vi "Read IL Action.vi"(11 "IL Action in":refnum<class "IL Action.lvclass">) -> (1 "Message Priority (Normal)":T1=enum."Normal", 3 "IL Action out":refnum<class "IL Action.lvclass">, 4 "Actor Framework:Message":refnum<class "Message.lvclass">, 5 "Action Destination":refnum<class "Message Enqueuer.lvclass">)   [LabVIEW 2015, in "Interlocks.lvlib" / "IL Action.lvclass"]
uses:
  IL Action.lvclass
  <vilib>/ActorFramework/Message/Message.lvclass
  <vilib>/ActorFramework/Message Enqueuer/Message Enqueuer.lvclass
  <vilib>/ActorFramework/Message Enqueuer/Message Priority.ctl
  IL Action.lvclass/IL Action.ctl
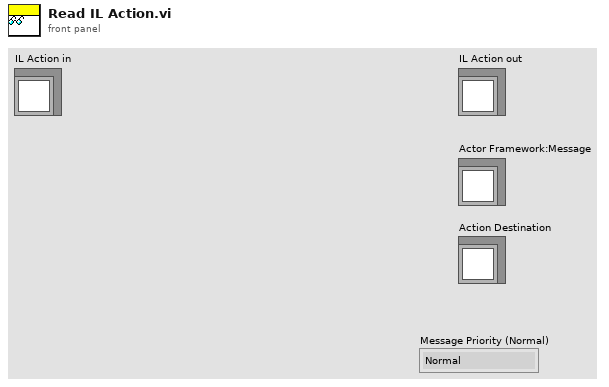
[diagram p1: front panel]
types:
  T1 = typedef "Actor Framework.lvlib/Message Enqueuer.lvclass/Message Priority.ctl" = enum16{"Low", "Normal", "High"}
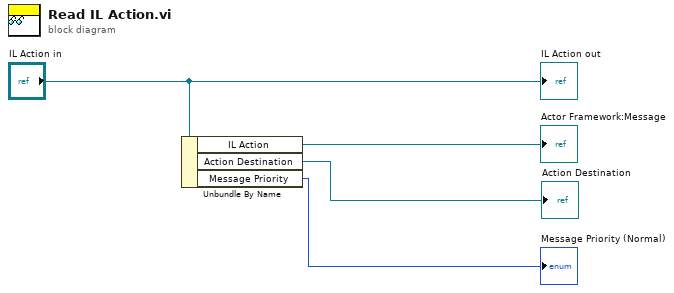
[diagram p0: block diagram]
diagram:
  n1 = Unbundle By Name("IL Action in") -> ("IL Action"=→"Actor Framework:Message":refnum<class "Message.lvclass">, "Action Destination"=→"Action Destination":refnum<class "Message Enqueuer.lvclass">, "Message Priority"=→"Message Priority (Normal)":T1)
  "IL Action out" <- "IL Action in"
